vi "(SubVI) Extract description CB.vi"(1 "Talent 2":string, 2 "Talent 1":string, 3 "Talent order CB":string[](array[string]), 4 "arr Description CB":string[](array[string])) -> (0 "Description CB":string)   [LabVIEW 2024]
panel:
  out "idx":i32
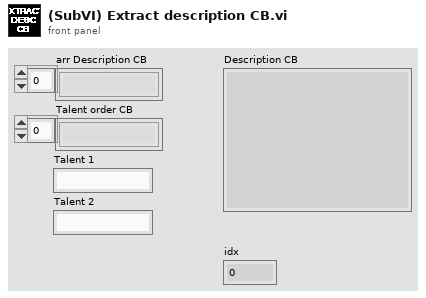
[diagram p1: front panel]
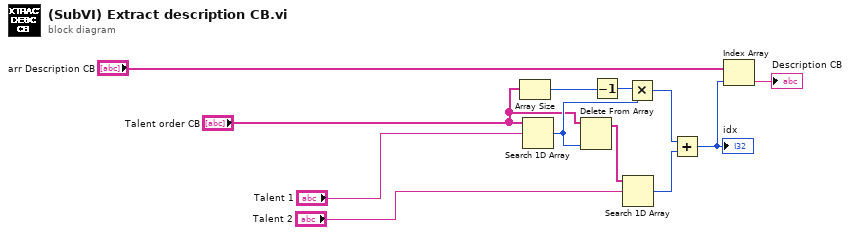
[diagram p0: block diagram]
diagram:
  n1 = Array Size(array="Talent order CB") -> (size(s)=w5:i32)
  n2 = Search 1D Array(1D array="Talent order CB", element="Talent 1") -> (index of element=w6:i32)  [unwired: 1 in]
  n3 = Delete From Array(array="Talent order CB", index=w6) -> (array with subset deleted=w2:string[])  [unwired: 1 in, 1 out]
  n4 = Decrement(x=w5) -> (x-1=w9:i32)
  n5 = Search 1D Array(1D array=w2, element="Talent 2") -> (index of element=w8:i32)  [unwired: 1 in]
  n6 = Multiply(x=w9, y=w6) -> (x*y=w7:i32)
  n7 = Add(x=w7, y=w8) -> (x+y=w11:i32)
  "idx" <- w11
  n8 = Index Array(array="arr Description CB", index=w11) -> (element=→"Description CB":string)
